vi "Send connect_to_hydraharp.vi"(4 "update_hydraharp_status":refnum<user-event>, 6 "ui_events":T1, 7 "Message Priority (Normal)":T7=enum."Normal", 8 "error in (no error)":errorcluster, 9 "Mode":T2 items=["T2"=2, "T3"=3], 10 "Hydraharp Settings":T3 {"CH 8"."ch_offs" min=-99999 max=99999 step=1; "CH 8"."ch_ZeroX" min=0 max=20 step=1; "CH 8"."ch_level" min=0 max=800 step=1; "CH 7"."ch_offs" min=-99999 max=99999 step=1; "CH 7"."ch_ZeroX" min=0 max=20 step=1; "CH 7"."ch_level" min=0 max=800 step=1; "CH 6"."ch_offs" min=-99999 max=99999 step=1; "CH 6"."ch_ZeroX" min=0 max=20 step=1; "CH 6"."ch_level" min=0 max=800 step=1; "CH 5"."ch_offs" min=-99999 max=99999 step=1; "CH 5"."ch_ZeroX" min=0 max=20 step=1; "CH 5"."ch_level" min=0 max=800 step=1; "binning" min=0 max=10 step=1; "CH 4"."ch_offs" min=-99999 max=99999 step=1; "CH 4"."ch_ZeroX" min=0 max=20 step=1; "CH 4"."ch_level" min=0 max=800 step=1; "CH 3"."ch_offs" min=-99999 max=99999 step=1; "CH 3"."ch_ZeroX" min=0 max=20 step=1; "CH 3"."ch_level" min=0 max=800 step=1; "CH 2"."ch_offs" min=-99999 max=99999 step=1; "CH 2"."ch_ZeroX" min=0 max=20 step=1; "CH 2"."ch_level" min=0 max=800 step=1; "CH 1"."ch_offs" min=-99999 max=99999 step=1; "CH 1"."ch_ZeroX" min=0 max=20 step=1; "CH 1"."ch_level" min=0 max=800 step=1; "Sync Settings"."snc_offs" min=-99999 max=99999 step=1; "Sync Settings"."snc_ZeroX" min=0 max=20 step=1; "Sync Settings"."snc_level" min=0 max=800 step=10}, 11 "Message Enqueuer":refnum<class "Message Enqueuer.lvclass">) -> (0 "error out":errorcluster, 3 "Message Enqueuer out":refnum<class "Message Enqueuer.lvclass">)   [LabVIEW 2015, in "connect_to_hydraharp Msg.lvclass"]
doc: "This VI sends the message to an actor."
uses:
  connect_to_hydraharp Msg.lvclass
  <vilib>/ActorFramework/Message Enqueuer/Message Enqueuer.lvclass
  <vilib>/ActorFramework/Message Enqueuer/Message Priority.ctl
  hydraharp_panel/hpanel_hydraharp_settings.ctl
  hydraharp_panel/hpanel_sync_settings.ctl
  hydraharp_panel/hpanel_sync_div.ctl
  hydraharp_panel/hpanel_channel_settings.ctl
  hydraharp_panel/hpanel_acq_modes.ctl
  UI/front_panel_class/ui_user_events.ctl
  connect_to_hydraharp Msg.lvclass/connect_to_hydraharp Msg.ctl
  <vilib>/ActorFramework/Message Enqueuer/Message Enqueuer.lvclass/Message Enqueuer.ctl
  <vilib>/ActorFramework/Message Priority Queue/Priority Enqueue.vi
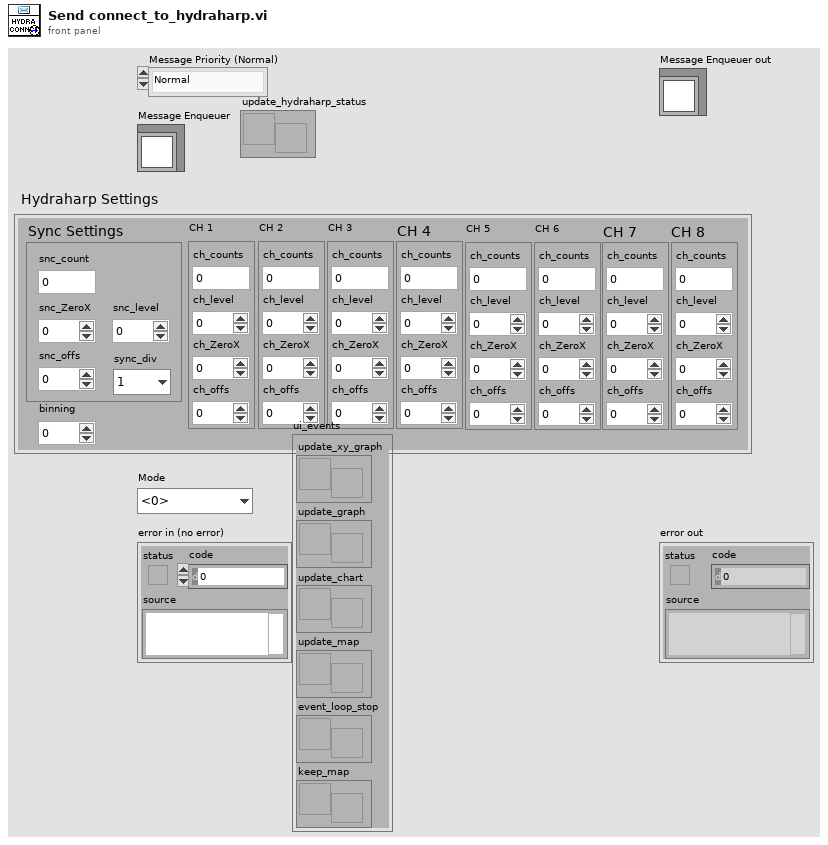
[diagram p1: front panel]
types:
  T1 = typedef "ui_user_events.ctl" = cluster{"update_xy_graph":refnum<user-event>, "update_graph":refnum<user-event>, "update_chart":refnum<user-event>, "update_map":refnum<user-event>, "event_loop_stop":refnum<user-event>, "keep_map":refnum<user-event>}
  T2 = typedef "hpanel_acq_modes.ctl" = u16
  T3 = typedef "hpanel_hydraharp_settings.ctl" = cluster{"Sync Settings":T4, "CH 1":T6, "CH 2":T6, "CH 3":T6, "CH 4":T6, "binning":i32, "CH 5":T6, "CH 6":T6, "CH 7":T6, "CH 8":T6}
  T4 = typedef "hpanel_sync_settings.ctl" = cluster{"snc_count":i32, "snc_level":i32, "snc_ZeroX":i32, "snc_offs":i32, "sync_div":T5}
  T5 = typedef "hpanel_sync_div.ctl" = enum16{"1", "2", "4", "8"}
  T6 = typedef "hpanel_channel_settings.ctl" = cluster{"ch_counts":i32, "ch_level":i32, "ch_ZeroX":i32, "ch_offs":i32}
  T7 = typedef "Actor Framework.lvlib/Message Enqueuer.lvclass/Message Priority.ctl" = enum16{"Low", "Normal", "High"}
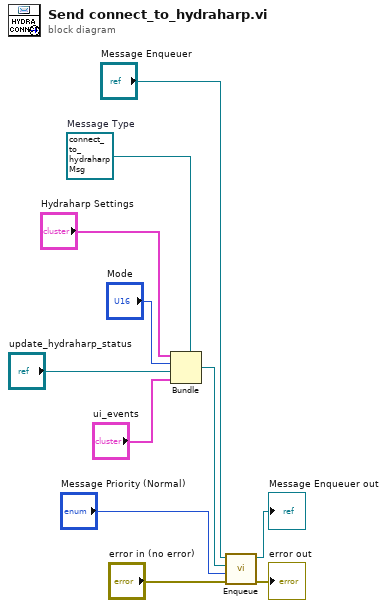
[diagram p0: block diagram]
diagram:
  w8 = refnum<class "connect_to_hydraharp Msg.lvclass"> refnum  # Message Type
  n1 = Bundle(cluster=w8, "Hydraharp Settings", "Mode", "update_hydraharp_status", "ui_events") -> (w7:refnum<class "connect_to_hydraharp Msg.lvclass">)
  n2 = call <vilib>:"Enqueue.vi"("error in (no error)"="error in (no error)", "Message Priority (Normal)"="Message Priority (Normal)", "Message"=w7, "Message Enqueuer in"="Message Enqueuer") -> ("error out"=→"error out":errorcluster, "Message Enqueuer out"=→"Message Enqueuer out":refnum<class "Message Enqueuer.lvclass">)  [unwired: 6 in]
